vi "Configure Arbitrary Waveform.vi"   [LabVIEW 2019, in "Agilent N7976A.lvlib"]
doc: "Polymorphic VI allows the selection between an arbitrary voltage waveform and an arbitrary current waveform."
uses:
  <instrlib>/Agilent N7976A/Agilent N7976A.lvlib
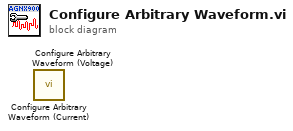
[diagram p0: block diagram]
diagram:
  n1 = call <instrlib>:"Configure Arbitrary Waveform (Current).vi"() -> ()  [unwired: 10 in, 2 out]
  n2 = call <instrlib>:"Configure Arbitrary Waveform (Voltage).vi"() -> ()  [unwired: 10 in, 2 out]
